vi "Set 项标识符.vi"(10 "项标识符":string, 11 "LNK in":refnum<class "Menu.lvclass">) -> (3 "LNK out":refnum<class "Menu.lvclass">)   [LabVIEW 2016, in "Menu.lvclass"]
uses:
  Menu.lvclass
  Menu.lvclass/Menu.ctl
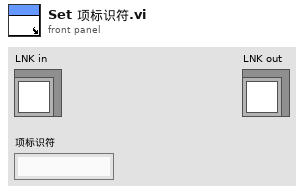
[diagram p1: front panel]
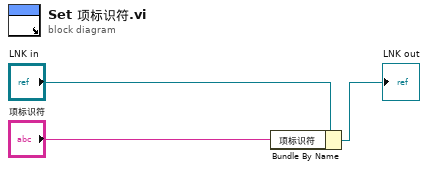
[diagram p0: block diagram]
diagram:
  n1 = Bundle By Name(cluster="LNK in", "项标识符"="项标识符") -> (→"LNK out":refnum<class "Menu.lvclass">)
